vi "TestMoteComm.vi"() -> ()   [LabVIEW 2010]
uses:
  <vilib>/picture/picture.llb/Draw True-Color Pixmap.vi
panel:
  out "Counter Send/receive":dynamicdata(graph)
  out "Bytes written":i32
  out "Packet Sent":string
  in  "Enable Write":bool=TRUE
  out "bytes read":i32
  out "Packet Payload":string
  in  "Enable Read":bool=TRUE
  in  "Port Number":i32=9002
  out "KTH  Automatic Control \nTemplates. Test Bi-directional communication \nSerialForwarder-Mote":picture
  # "WRITE PACKET"
  # "READ PACKET"
  # "For TestSerialCommMsg:\nheaderSize = 9\npayload = 4"
  # "Communication control"
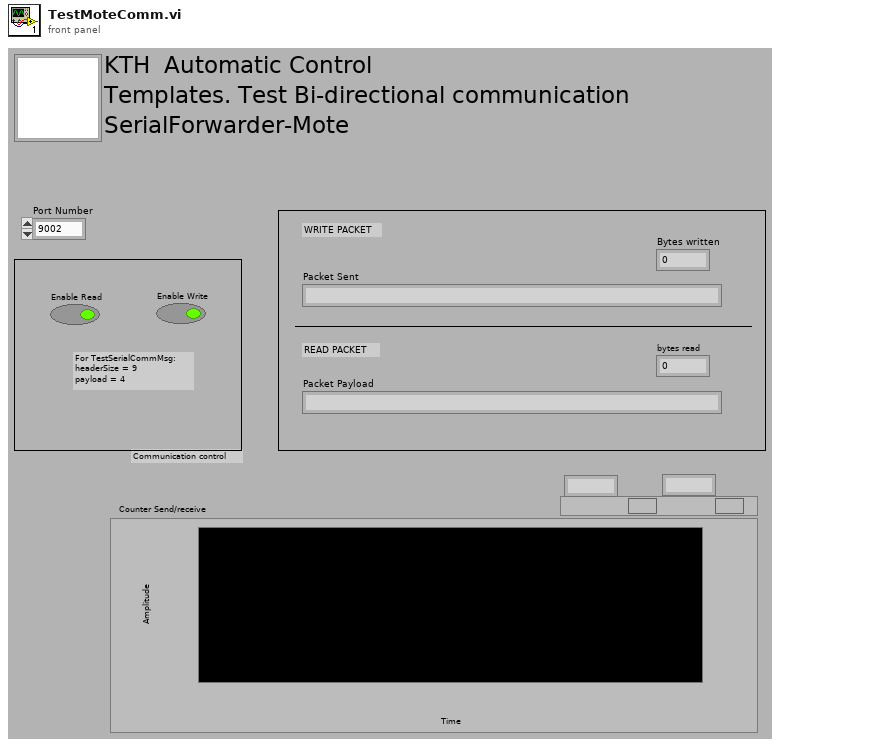
[diagram p1: front panel]
types:
  T1 = typedef "imagedata.ctl" = cluster{"image type":i32, "image depth":i32, "image":u8[], "mask":u8[], "colors":u32[], "Rectangle":cluster{"left":i16, "top":i16, "right":i16, "bottom":i16}}
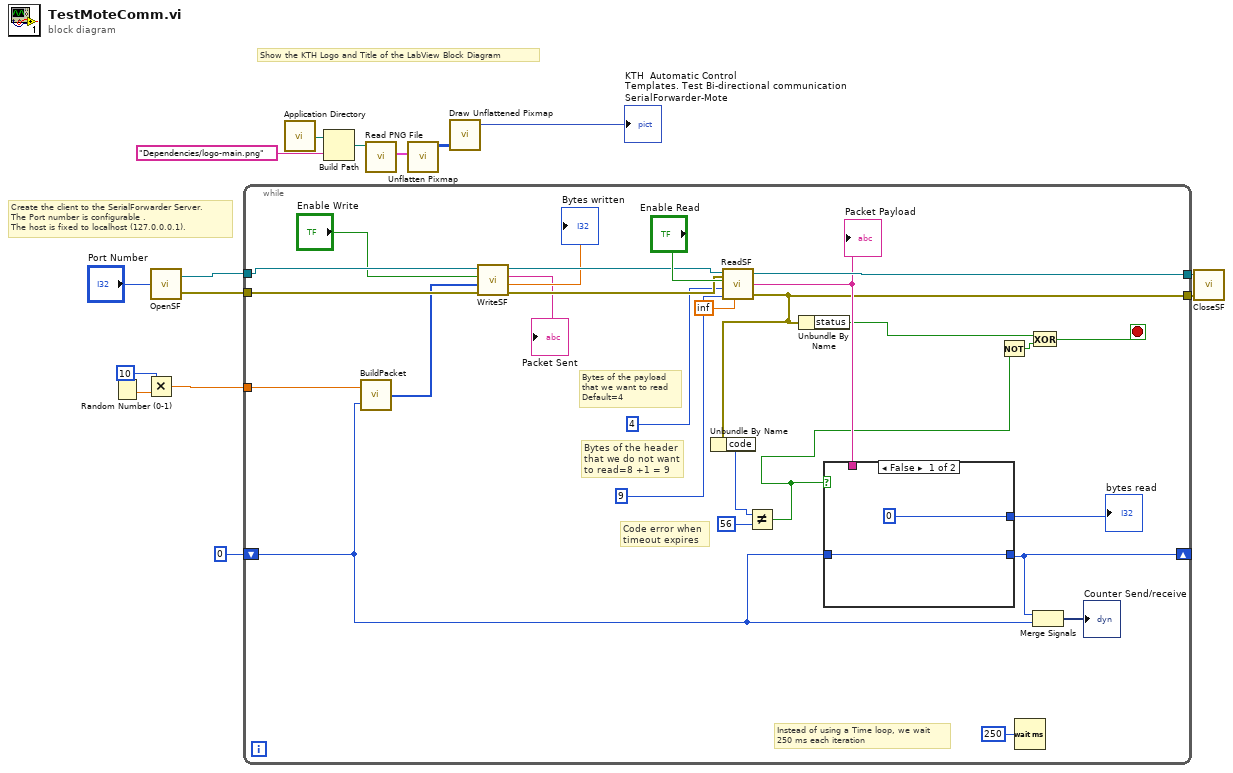
[diagram p0: block diagram]
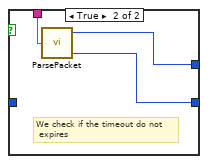
[diagram p2: hidden frame]
diagram:
  # "Create the client to the SerialForwarder Server.\nThe Port number is configurable . \nThe host is fixed to localhost (127.0.0.0.1)."
  # "Show the KTH Logo and Title of the LabView Block Diagram"
  n1 = Random Number (0-1)() -> (number: 0 to 1=w3:dbl)
  n2 = Multiply(x=u16 10, y=w3) -> (x*y=w1:dbl)
  n3 = call "OpenSF.vi"("Port Number"="Port Number") -> ("error out"=w14:errorcluster, "connection ID"=w15:refnum<k5>)
  n4 = while {
    tunnel: w15 -> [w38]
    tunnel: w14 -> [w39]
    tunnel: [w42] -> w13
    tunnel: [w25] -> w12
    tunnel: w1 -> [w33]
    shift-right: [w27] -> _
    shift-left: u16 0 -> [w20]
    stop <- w21 stop-if-true
    # "Code error when  \ntimeout expires"
    # "Instead of using a Time loop, we wait \n250 ms each iteration"
    # "Bytes of the payload \nthat we want to read\nDefault=4"
    # "Bytes of the header\nthat we do not want \nto read=8 +1 = 9"
    n5 = call "BuildPacket.vi"("Counter"=w20, "Dummy"=w33) -> ("PacketArray"=w34:i32[])
    n6 = call "WriteSF.vi"("error in"=w39, "packet"=w34, "Enablle write"="Enable Write", "connection ID"=w38) -> ("error out"=w36:errorcluster, "Bytes written to SF"=→"Bytes written":dbl, "Packet String"=→"Packet Sent":string, "connection ID out"=w37:refnum<k5>)
    n7 = call "ReadSF.vi"("connection ID in"=w37, "error in"=w36, "enabled"="Enable Read", "bytes to read"=4, "timeout (optional)"=inf, "header size"=9 ("bytes to read")) -> ("connection ID out"=w42:refnum<k5>, "string"=w40:string, "error out"=w25:errorcluster)
    "Packet Payload" <- w40
    n8 = Unbundle By Name(w25) -> ("code"=w24:i32)
    n9 = Not Equal?(x=w24, y=56) -> (x != y?=w16:bool)
    n10 = Unbundle By Name(w25) -> ("status"=w22:bool)
    n11 = case shown="False" w16 {
      tunnel: w40 -> [_ w47]
      tunnel: [0 ("Bytes read") w46] -> w19
      tunnel: [w44 w45] -> w27
      tunnel: w20 -> [w44 _]
      frame False {
      }
      frame True {
        # "We check if the timeout do not\n expires"
        n12 = call "ParsePacket.vi"("data out"=w47) -> ("Counter"=w45:i16, "Bytes read"=w46:i32)  [unwired: 1 out]
      }
    }
    "bytes read" <- w19
    n13 = Not(x=w16) -> (.not. x?=w17:bool)
    n14 = Wait (ms)(milliseconds to wait=u32 250) -> ()  [unwired: 1 out]
    n15 = Exclusive Or(1:w17, 2:w22) -> (0:w21:bool)
    n16 = Merge Signals(w27, w20) -> (→"Counter Send/receive":dynamicdata)
  }
  n17 = call <vilib>:"Application Directory.vi"() -> ("Application Directory"=w7:path)
  n18 = Build Path(base path=w7, name or relative path="Dependencies/logo-main.png") -> (appended path=w8:path)
  n19 = call <vilib>:"Read PNG File.vi"("path to PNG file"=w8) -> ("image data"=w11:T1)  [unwired: 8 in, 2 out]
  n20 = call <vilib>:"Unflatten Pixmap.vi"("image data"=w11) -> ("24-bit pixmap"=w10:u32[][])  [unwired: 4 in, 6 out]
  n21 = call-poly <vilib>:"Draw Unflattened Pixmap.vi"("data (RGB format)"=w10) -> ("new picture"=→"KTH  Automatic Control \nTemplates. Test Bi-directional communication \nSerialForwarder-Mote":picture)  [unwired: 8 in]
  n22 = call "CloseSF.vi"("error out"=w12, "connection ID"=w13) -> ()  [unwired: 1 in]
